vi "main_clear_environment.vi"(5 "Flow":refnum<vi>, 6 "Env. Clear":refnum<vi>, 7 "Running?":refnum<vi>, 8 "Starttime":refnum<vi>, 9 "Env. ready?":refnum<vi>, 10 "Env. Dir":refnum<vi>, 11 "Env. Tree":refnum<vi>) -> ()   [LabVIEW 2019]
panel:
  # "*******************************************************************\nBiogas Plant Control\n\nAuthor: Paul Zügel\nGCSC-Frankfurt am Main 2020\n\n*******************************************************************"
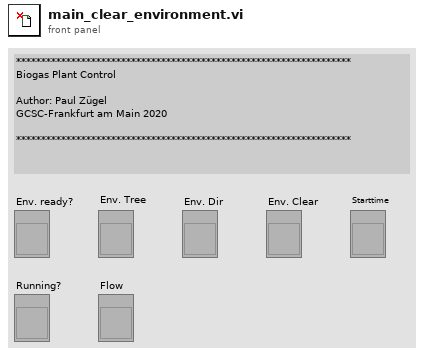
[diagram p1: front panel]
types:
  T1 = enum8{"Enabled", "Disabled", "Disabled and Grayed Out"}
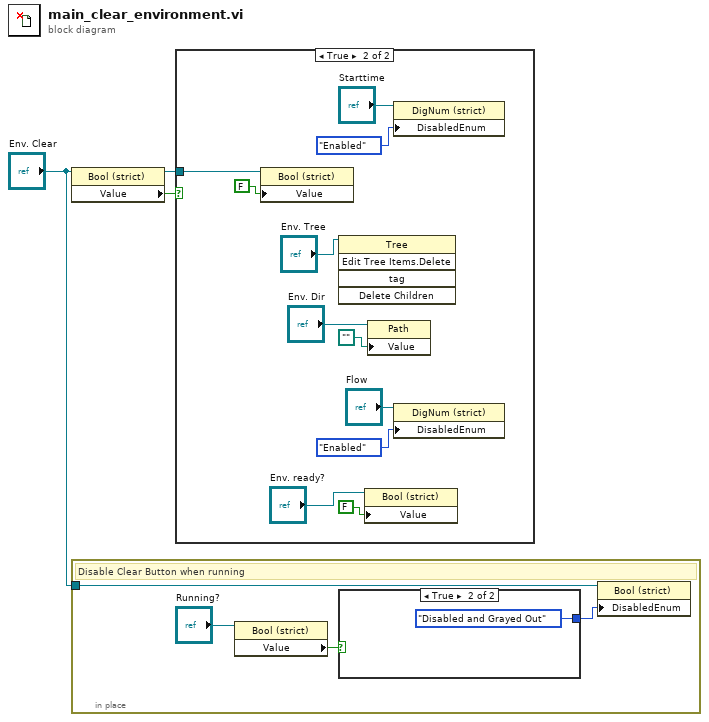
[diagram p0: block diagram]
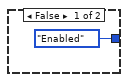
[diagram p2: hidden frame]
diagram:
  n1 = property class="Bool (strict)"(reference="Env. Clear") -> (reference out=w2:refnum<vi>, "Value"=w3:bool)  [unwired: 1 in, 1 out]
  n2 = in-place {
    in-place-border: "Env. Clear" -> [w5]
    # "Disable Clear Button when running"
    n3 = property class="Bool (strict)"(reference="Running?") -> ("Value"=w6:bool)  [unwired: 1 in, 2 out]
    n4 = case shown="True" w6 {
      tunnel: [T1."Enabled" ("Disabled") T1."Disabled and Grayed Out" ("Disabled")] -> w4
      frame False {
      }
      frame True {
      }
    }
    n5 = property class="Bool (strict)"(reference=w5, "DisabledEnum"=w4) -> ()  [unwired: 1 in, 2 out]
  }
  n6 = case shown="True" w3 {
    tunnel: w2 -> [_ w20]
    frame False {
    }
    frame True {
      n7 = property class="Bool (strict)"(reference=w20, "Value"=FALSE) -> ()  [unwired: 1 in, 2 out]
      n8 = invoke class="Tree" method="Edit Tree Items.Delete"(reference="Env. Tree") -> ()  [unwired: 4 in, 5 out]
      n9 = property class="Bool (strict)"(reference="Env. ready?", "Value"=FALSE) -> ()  [unwired: 1 in, 2 out]
      n10 = property class="Path"(reference="Env. Dir", "Value"=path "") -> ()  [unwired: 1 in, 2 out]
      n11 = property on="Property Node" class="DigNum (strict)"(reference="Starttime", "DisabledEnum"=T1."Enabled" ("Disabled")) -> ()  [unwired: 1 in, 2 out]
      n12 = property on="Property Node" class="DigNum (strict)"(reference="Flow", "DisabledEnum"=T1."Enabled" ("Disabled")) -> ()  [unwired: 1 in, 2 out]
    }
  }
